vi "Main Page.vi"(8 "error in (no error)":errorcluster, 11 "Node Ptr":T2 format="%.0x") -> (0 "error out":errorcluster)   [LabVIEW 2016, in "FPGA RM Test Custom Device System Explorer.lvlib"]
uses:
  FPGA RM Test Custom Device System Explorer.lvlib
  <vilib>/NI Veristand/Custom Device API/Custom Device Item Ref.ctl
  Source/RM.clientInfo.ctl
  Source/RM.resourceType.ctl
  <vilib>/NI Veristand/Custom Device API/Custom Device API.lvlib
  Source/FPGA Resource Manager.lvlib
panel:
  in  "Server GUID":string
  in  "name in bitfile":string
  out "ClientInfo Array":T1[](array[typedef]) {"CD Ref" format="%.0x"}
  in  "Reserve Scalar Output":bool
  in  "Header":cluster{"Section Name":string}={"Section Name"="Custom Device Item Settings"}
  in  "Description":string
  in  "Name":string
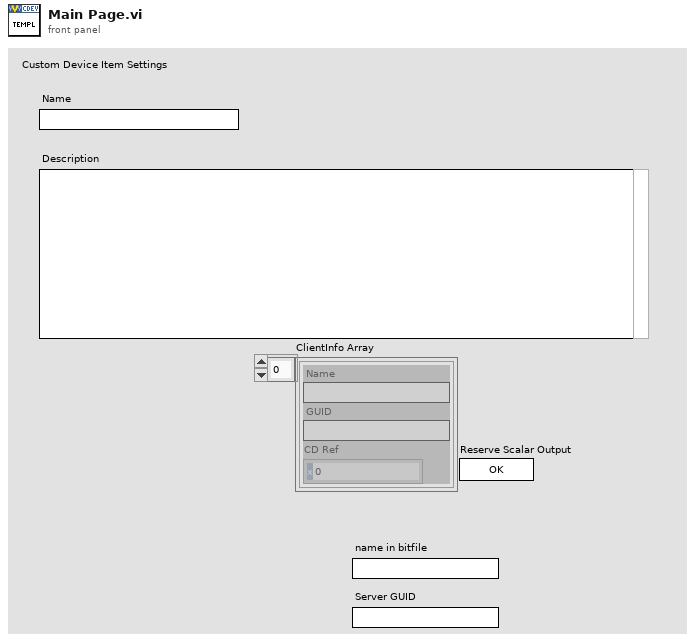
[diagram p1: front panel]
types:
  T1 = typedef "FPGA Resource Manager.lvlib/RM.clientInfo.ctl" = cluster{"Name":string, "GUID":string, "CD Ref":T2}
  T2 = typedef "Custom Device API.lvlib/Custom Device Item Ref.ctl" = u64
  T3 = typedef "Custom Device API.lvlib/Custom Device Item Info.ctl" = cluster{"Name":string, "Is Channel":bool, "GUID":string, "Is Waveform":bool}
  T4 = typedef "FPGA Resource Manager.lvlib/RM.resourceType.ctl" = enum16{"Scalar Input", "Scalar Output", "Waveform Input", "Waveform Output"}
  T5 = typedef "Custom Device API.lvlib/Custom Device Commands.ctl" = enum16{"Default", "Item renamed", "Shutdown", "Dynamic button pressed"}
  T6 = typedef "FPGA Resource Manager.lvlib/RM.serverInfo.ctl" = cluster{"name":string, "guid":string, "cd node ref":T2, "database":variant}
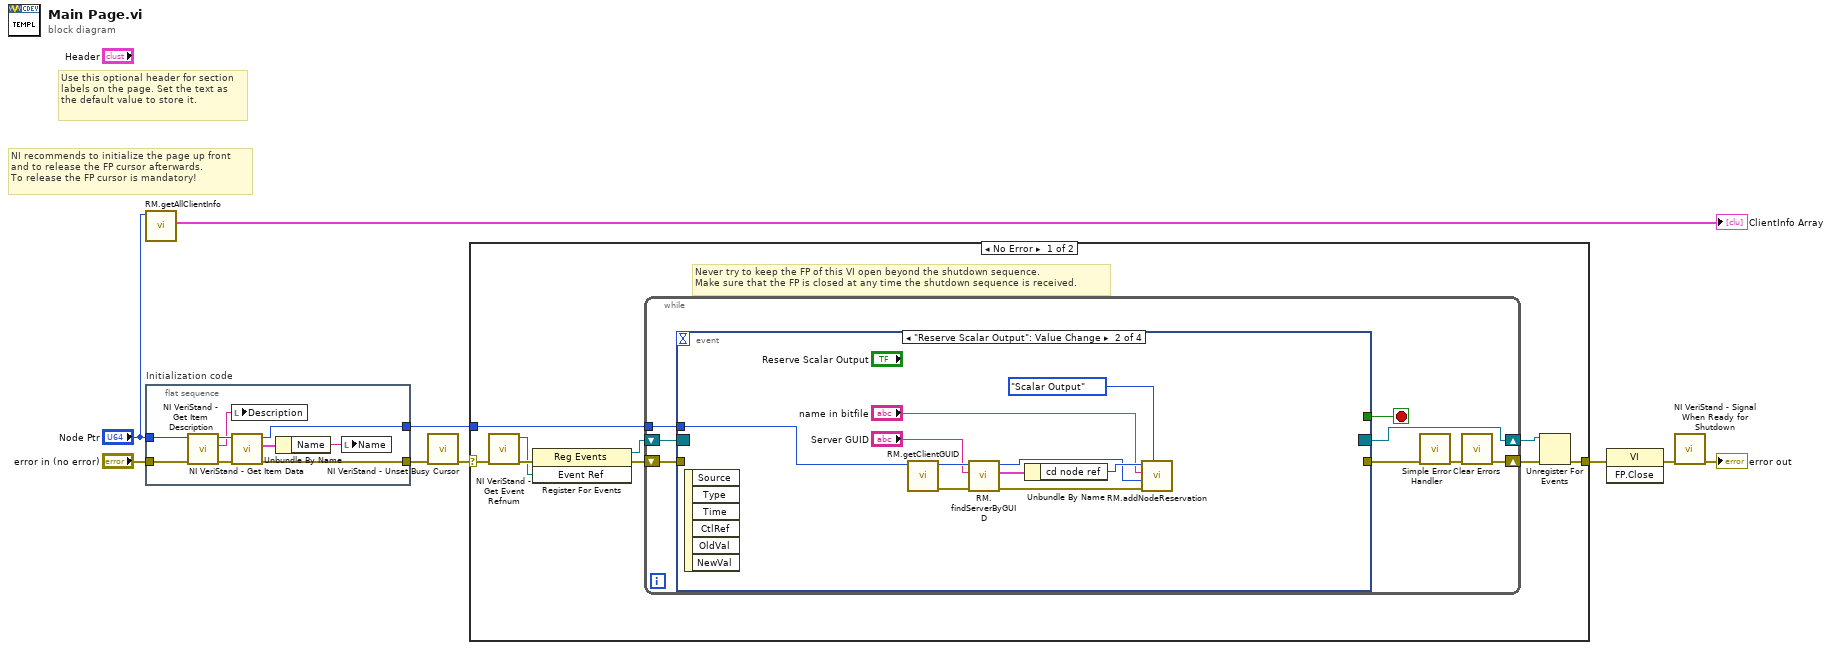
[diagram p0: block diagram]
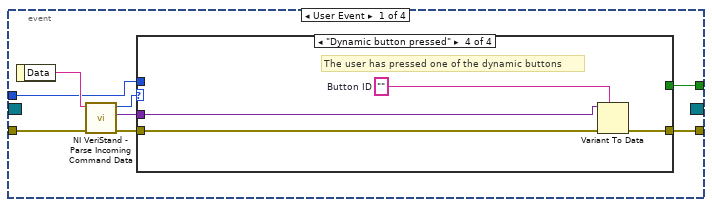
[diagram p2: hidden frame]
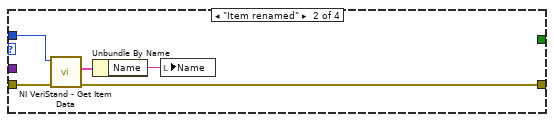
[diagram p4: hidden frame]
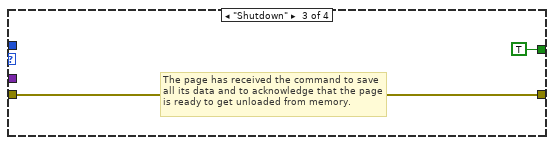
[diagram p5: hidden frame]
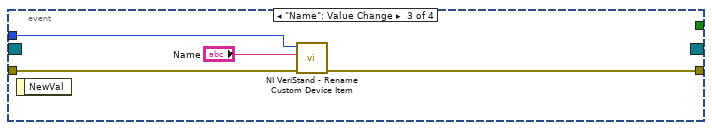
[diagram p6: hidden frame]
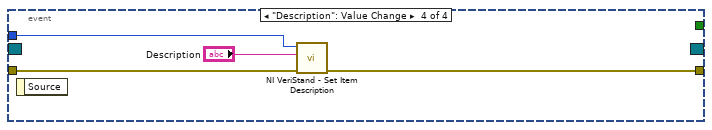
[diagram p7: hidden frame]
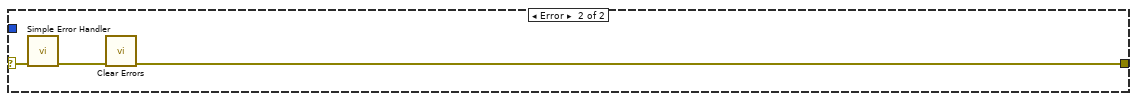
[diagram p8: hidden frame]
diagram:
  # "Use this optional header for section labels on the page. Set the text as the default value to store it."
  # "NI recommends to initialize the page up front\nand to release the FP cursor afterwards.\nTo release the FP cursor is mandatory!"
  n1 = call "RM.getAllClientInfo.vi"("Item Ref in"="Node Ptr") -> ("ClientInfo Array"=→"ClientInfo Array":T1[])  [unwired: 8 in, 2 out]
  n2 = flat-sequence "Initialization code" {
    tunnel: "error in (no error)" -> [w16]
    tunnel: "Node Ptr" -> [w15]
    tunnel: [w10] -> w6
    tunnel: [w18] -> w3
    frame #0 {
      n3 = call <vilib>:"NI VeriStand - Get Item Description.vi"("error in (no error)"=w16, "Item Ref in"=w15) -> ("error out"=w13:errorcluster, "Description"=w14:string, "Item Ref out"=w17:T2)  [unwired: 7 out]
      n4 = local write "Description"(w14) -> ()
      n5 = call <vilib>:"NI VeriStand - Get Item Data.vi"("error in (no error)"=w13, "Item Ref in"=w17) -> ("error out"=w10:errorcluster, "Item Info"=w12:T3, "Item Ref out"=w18:T2)  [unwired: 7 out]
      n6 = Unbundle By Name(w12) -> ("Name"=w11:string)
      n7 = local write "Name"(w11) -> ()
    }
  }
  n8 = call <vilib>:"NI VeriStand - Unset Busy Cursor.vi"("error in (no error)"=w6) -> ("error out"=w5:errorcluster)  [unwired: 10 out]
  n9 = case shown="No Error" w5 {
    selector: w5 -> [w19 w76]
    tunnel: [w24 w74] -> w9
    tunnel: w3 -> [w20 _]
    frame No Error {
      # "Never try to keep the FP of this VI open beyond the shutdown sequence.\nMake sure that the FP is closed at any time the shutdown sequence is received."
      n10 = call <vilib>:"NI VeriStand - Get Event Refnum.vi"("error in (no error)"=w19) -> ("error out"=w27:errorcluster, "Event Ref"=w23:refnum<user-event>)  [unwired: 9 out]
      n11 = register-events(error in=w27, w23) -> (reference out=w21:refnum<event-registration>, error out=w22:errorcluster)  [unwired: 1 in]
      n12 = while {
        tunnel: w20 -> [w31]
        shift-right: [w28] -> w25
        shift-left: w22 -> [w34]
        shift-right: [w35] -> w26
        shift-left: w21 -> [w33]
        stop <- w32 stop-if-true
        n13 = event shown="[1] \"Reserve Scalar Output\": Value Change" {
          selector: w33 -> [_ _ _ _]
          dyn-events: [_ _ _ _] -> w35
          timeout: _ -> [_ _ _ _]
          tunnel: w34 -> [w43 _ w69 w72]
          tunnel: [w39 _ _ _] -> w32
          tunnel: [w38 _ w68 w71] -> w30
          tunnel: w31 -> [w37 w65 w67 w73]
          event User Event {
            n14 = event-data() -> ("Data"=w42:string)  [unwired: 1 out]
            n15 = call <vilib>:"NI VeriStand - Parse Incoming Command Data.vi"("error in (no error)"=w43, "Incoming data"=w42) -> ("error out"=w41:errorcluster, "Outgoing data"=w36:variant, "Action"=w40:T5)  [unwired: 7 out]
            n16 = case shown="\"Dynamic button pressed\"" w40 {
              tunnel: w41 -> [w44 w49 w50 w55]
              tunnel: [_ _ TRUE _] -> w39
              tunnel: [w44 w46 w50 w52] -> w38
              tunnel: w37 -> [_ w48 _ _]
              tunnel: w36 -> [_ _ _ w54]
              frame "Default", Default {
              }
              frame "Item renamed" {
                n17 = call <vilib>:"NI VeriStand - Get Item Data.vi"("error in (no error)"=w49, "Item Ref in"=w48) -> ("error out"=w46:errorcluster, "Item Info"=w47:T3)  [unwired: 8 out]
                n18 = Unbundle By Name(w47) -> ("Name"=w45:string)
                n19 = local write "Name"(w45) -> ()
              }
              frame "Shutdown" {
                # "The page has received the command to save all its data and to acknowledge that the page is ready to get unloaded from memory."
              }
              frame "Dynamic button pressed" {
                w53 = ""  # Button ID
                # "The user has pressed one of the dynamic buttons"
                n20 = Variant To Data(error in=w55, type=w53, Variant=w54) -> (error out=w52:errorcluster)  [unwired: 1 out]
              }
            }
          }
          event "Reserve Scalar Output": Value Change {
            n21 = event-data() -> ()  [unwired: 7 out]
            n22 = call "RM.getClientGUID.vi"("Item Ref in"=w65) -> ("error out"=w62:errorcluster, "Item Ref out"=w64:T2)  [unwired: 7 in, 2 out]
            n23 = call "RM.findServerByGUID.vi"("error in"=w62, "serverGUID"="Server GUID", "Item Ref in"=w64) -> ("error out"=w58:errorcluster, "serverInfo"=w61:T6, "Item Ref out"=w56:T2)  [unwired: 5 in, 1 out]
            n24 = Unbundle By Name(w61) -> ("cd node ref"=w60:T2)
            n25 = call "RM.addNodeReservation.vi"("Resource Type"=RM.resourceType."Scalar Output", "error in"=w58, "Server Ref in"=w56, "name in bitfile"="name in bitfile", "Client Ref In"=w60) -> ()  [unwired: 4 in, 3 out]
          }
          event "Name": Value Change {
            n26 = event-data() -> ()  [unwired: 2 out]
            n27 = call <vilib>:"NI VeriStand - Rename Custom Device Item.vi"("error in (no error)"=w69, "New Name"="Name", "Item Ref in"=w67) -> ("error out"=w68:errorcluster)  [unwired: 1 in, 7 out]
          }
          event "Description": Value Change {
            n28 = event-data() -> ()  [unwired: 2 out]
            n29 = call <vilib>:"NI VeriStand - Set Item Description.vi"("error in (no error)"=w72, "Description"="Description", "Item Ref in"=w73) -> ("error out"=w71:errorcluster)  [unwired: 8 out]
          }
        }
        n30 = call <vilib>:"Simple Error Handler.vi"("error in (no error)"=w30) -> ("error out"=w29:errorcluster)  [unwired: 1 in, 7 out]
        n31 = call <vilib>:"Clear Errors.vi"("error in (no error)"=w29) -> ("error out"=w28:errorcluster)  [unwired: 1 in, 5 out]
      }
      n32 = Unregister For Events(event registration refnum=w26, error in=w25) -> (error out=w24:errorcluster)
    }
    frame Error {
      n33 = call <vilib>:"Simple Error Handler.vi"("error in (no error)"=w76) -> ("error out"=w75:errorcluster)  [unwired: 1 in, 7 out]
      n34 = call <vilib>:"Clear Errors.vi"("error in (no error)"=w75) -> ("error out"=w74:errorcluster)  [unwired: 1 in, 5 out]
    }
  }
  n35 = invoke class="VI" method="FP.Close"(error in=w9) -> (error out=w8:errorcluster)  [unwired: 2 in, 2 out]
  n36 = call <vilib>:"NI VeriStand - Signal When Ready for Shutdown.vi"("error in (no error)"=w8) -> ("error out"=→"error out":errorcluster)  [unwired: 10 out]
